vi "Discovery UDP Receive Loop.vi"(0 "stop notifier":refnum<notifier>, 5 "discovered host queue":refnum<queue>, 9 "discoveryPort":u16=10001) -> (15 "error out":errorcluster)   [LabVIEW 2020, in "epl-network.lvlib"]
uses:
  epl-network.lvlib
  Discovered Host.ctl
  Public/Discovery/Typedefs/Server Beacon.ctl
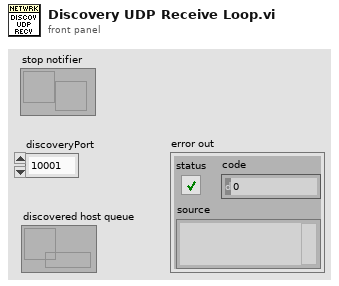
[diagram p1: front panel]
types:
  T1 = typedef "epl-network.lvlib/Server Beacon.ctl" = cluster{"name":string, "addr":string, "port":u16, "ver":u16}
  T2 = cluster{"DiscoveryBeacon":T1, "seconds since 1Jan1904":timestamp}
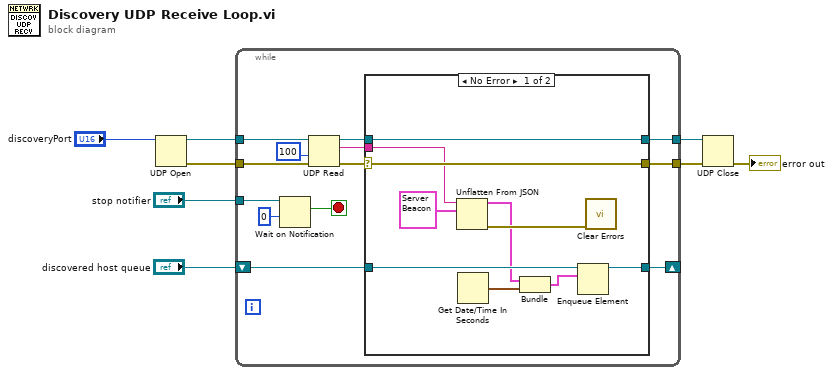
[diagram p0: block diagram]
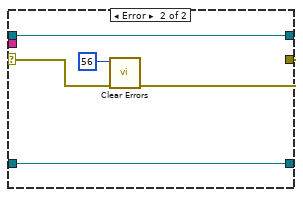
[diagram p2: hidden frame]
diagram:
  n1 = UDP Open(11:"discoveryPort") -> (port=w5:refnum<k16>, 0:w6:errorcluster)  [unwired: 4 in, 1 out]
  n2 = while {
    tunnel: w5 -> [w21]
    tunnel: w6 -> [w20]
    tunnel: [w19] -> w7
    tunnel: [w18] -> w8
    tunnel: "stop notifier" -> [w13]
    shift-right: [w11] -> _
    shift-left: "discovered host queue" -> [w12]
    stop <- w10 stop-if-true
    n3 = Wait on Notification(notifier=w13, timeout in ms (-1)=0) -> (notification=w10:bool)  [unwired: 2 in, 3 out]
    n4 = UDP Read(connection ID=w21, timeout ms (25000)=100, 8:w20) -> (data out=w15:string, error out=w16:errorcluster, 3:w14:refnum<k16>)  [unwired: 3 out]
    n5 = case shown="No Error" w16 {
      selector: w16 -> [w30 w36]
      tunnel: [w30 w34] -> w19
      tunnel: w15 -> [w29 _]
      tunnel: w14 -> [w31 w33]
      tunnel: [w31 w33] -> w18
      tunnel: w12 -> [w26 w32]
      tunnel: [w25 w32] -> w11
      frame No Error {
        n6 = Unflatten From JSON(JSON string=w29, type and defaults=T1 {"name"="", "addr"="192.168.1.98", "port"=57469, "ver"=10001} ("DiscoveryBeacon")) -> (value=w24:T1, error out=w27:errorcluster)  [unwired: 5 in]
        n7 = Get Date/Time In Seconds() -> (seconds since 1Jan1904=w23:timestamp)
        n8 = Bundle("DiscoveryBeacon"=w24, "seconds since 1Jan1904"=w23) -> (w22:T2)  [unwired: 1 in]
        n9 = Enqueue Element(queue=w26, element=w22) -> (queue out=w25:refnum<queue>)  [unwired: 2 in, 2 out]
        n10 = call <vilib>:"Clear Errors.vi"("error in (no error)"=w27) -> ()  [unwired: 5 in, 2 out]
      }
      frame Error {
        n11 = call <vilib>:"Clear Errors.vi"("error in (no error)"=w36, "specific error code to clear (0: all)"=56) -> ("error out"=w34:errorcluster)  [unwired: 4 in, 1 out]
      }
    }
  }
  n12 = UDP Close(connection ID=w8, 8:w7) -> (error out=→"error out":errorcluster)  [unwired: 1 out]
